vi "User Inputs.vi"() -> (3 "Operation States":T2)   [LabVIEW 2014]
uses:
  <vilib>/Rock Robotics/WPI/Solenoid/WPI_SolenoidValue.ctl
  <vilib>/Rock Robotics/WPI/Joystick/WPI_JoystickGetSetRefNum.vi
panel:
  out "Right Axis":dbl
  out "Left Axis":dbl
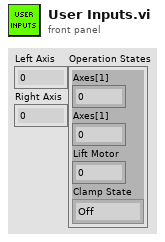
[diagram p1: front panel]
types:
  T1 = typedef "WPI_SolenoidValue.ctl" = enum16{"Off", "On", "Forward", "Reverse"}
  T2 = cluster{"Axes[1]":dbl, "Axes[1]":dbl, "Lift Motor":dbl, "Clamp State":T1}
  T3 = typedef "WPI_JoystickDevRef.ctl" = cluster{"Device":T4}
  T4 = typedef "WPI_JoystickDeviceEnum.ctl" = enum16{"USB 0", "USB 1", "USB 2", "USB 3", "USB 4", "USB 5"}
  T5 = cluster{"Buttons[0]":bool, "Buttons[1]":bool, "Buttons[2]":bool, "Buttons[3]":bool, "Buttons[4]":bool, "Buttons[5]":bool, "Buttons[6]":bool, "Buttons[7]":bool, "Buttons[8]":bool}
  T6 = cluster{"Axes[0]":dbl, "Axes[1]":dbl, "Axes[2]":dbl, "Axes[3]":dbl, "Axes[4]":dbl, "Axes[5]":dbl, "Axes[6]":dbl, "Axes[7]":dbl, "Axes[8]":dbl}
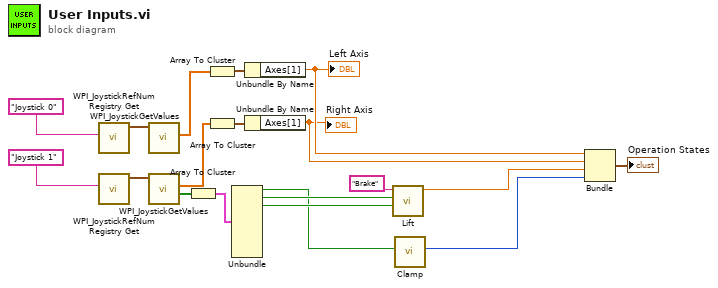
[diagram p0: block diagram]
diagram:
  n1 = call <vilib>:"WPI_JoystickRefNum Registry Get.vi"("refnum name"="Joystick 0") -> ("JoystickDevRef"=w18:T3)  [unwired: 1 in, 9 out]
  n2 = call <vilib>:"WPI_JoystickRefNum Registry Get.vi"("refnum name"="Joystick 1") -> ("JoystickDevRef"=w16:T3)  [unwired: 1 in, 9 out]
  n3 = call <vilib>:"WPI_JoystickGetValues.vi"("JoystickDevRef"=w18) -> ("Axes"=w12:dbl[])  [unwired: 6 in, 4 out]
  n4 = call <vilib>:"WPI_JoystickGetValues.vi"("JoystickDevRef"=w16) -> ("Buttons"=w15:bool[], "Axes"=w13:dbl[])  [unwired: 6 in, 3 out]
  n5 = Array To Cluster(array=w15) -> (cluster=w14:T5)
  n6 = Array To Cluster(array=w12) -> (cluster=w11:T6)
  n7 = Array To Cluster(array=w13) -> (cluster=w10:T6)
  n8 = Unbundle(w14) -> ("Buttons[0]"=w3:bool, "Buttons[1]"=w7:bool, "Buttons[2]"=w6:bool)  [unwired: 6 out]
  n9 = Unbundle By Name(w11) -> ("Axes[1]"=w9:dbl)
  "Left Axis" <- w9
  n10 = Unbundle By Name(w10) -> ("Axes[1]"=w8:dbl)
  "Right Axis" <- w8
  n11 = call "Lift.vi"("Up Button"=w6, "Down Button"=w7, "Solenoid Ref Name"="Brake") -> ("Lift Motor"=w5:dbl)  [unwired: 8 in]
  n12 = call "Clamp.vi"("Button"=w3) -> ("Clamp State"=w2:T1)  [unwired: 10 in]
  n13 = Bundle("Axes[1]"=w9, "Axes[1]"=w8, "Lift Motor"=w5, "Clamp State"=w2) -> (→"Operation States":T2)  [unwired: 1 in]
